vi "Test FPGA.vi"() -> ()   [LabVIEW 2014]
uses:
  <vilib>/FPGAPlugInAG/PXI-7842R/niLvFpga_Open_PXI-7842R.vi
  <vilib>/rvi/interface/common/dynamic/niFpgaDynamicAddResources.vi
  <vilib>/rvi/interface/common/niFpgaWaitOnOcc.vi
  <vilib>/Utility/error.llb/Error Cluster From Error Code.vi
  <vilib>/rvi/errors/niLvFpgaAdjustHostInterfaceError.vi
  <vilib>/RVI Host/nirviSupport.llb/nirviErrorClusterFromErrorCode.vi
  <vilib>/FPGAPlugInAG/Dynamic/niLvFpga_Close_Dynamic.vi
  <vilib>/rvi/interface/nirviOpenFPGA/nirviOpenFPGA.xnode
  FPGA Bitfiles/FPGA Server.lvbitx
  <vilib>/rvi/interface/nirviMethod/nirviMethod.xnode
  <vilib>/rvi/interface/nirviReadWriteControl/nirviReadWriteControl.xnode
  <vilib>/rvi/interface/nirviCloseFPGA/nirviCloseFPGA.xnode
  <vilib>/FPGAPlugInAG/Dynamic/niLvFpga_ConfigureFifo_Dynamic.vi
  <vilib>/rvi/errors/niLvFpgaMergeErrorWithErrorCode.vi
  NiFpgaLv.dll
  <vilib>/rvi/interface/Simulation/niFpgaSimulationCallBeginRW.vi
  <vilib>/FPGAPlugInAG/Dynamic/niLvFpga_StartFifo_Dynamic.vi
  <vilib>/FPGAPlugInAG/Dynamic/niLvFpga_WriteFifo_Dynamic.vi
  <vilib>/FPGAPlugInAG/Dynamic/niLvFpga_ReadFifo_Dynamic.vi
  <vilib>/rvi/interface/nirviMethod/StockFPGA_InlinedMethodWaitForSingleIRQ.vi
  <vilib>/FPGAPlugInAG/Dynamic/niLvFpga_WaitOnIrq_Dynamic.vi
  <vilib>/FPGAPlugInAG/Dynamic/niLvFpga_AcknowledgeIrq_Dynamic.vi
panel:
  in  "iSpk Enable":T1
  in  "LaserEn":T1
  out "Waveform Graph":i16[](graph)
  in  "Speaker":cluster{"Voltage":fxp<+,32,0>, "Offset":i16} {"Voltage" format="%.32g"}
  out "error out 2":errorcluster
  out "error out":errorcluster
  out "current time":timestamp
  out "Elements Remaining":u32
  in  "f0":i16=1350
  in  "Df":i16=200
  in  "Spk Enable":bool
  in  "Cell 5":T2 {"f0" format="%.32g"; "Scale" format="%.32g"}
  in  "Stop Button":bool
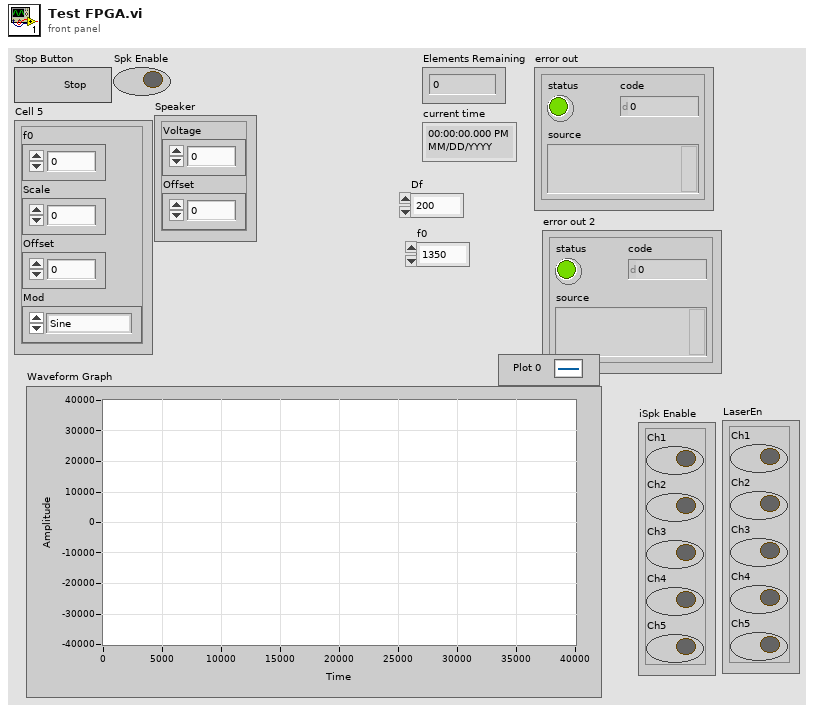
[diagram p1: front panel]
types:
  T1 = cluster{"Ch1":bool, "Ch2":bool, "Ch3":bool, "Ch4":bool, "Ch5":bool}
  T2 = cluster{"f0":fxp<+,32,0>, "Scale":fxp<+,32,0>, "Offset":i16, "Mod":enum8{"Sine", "Square"}}
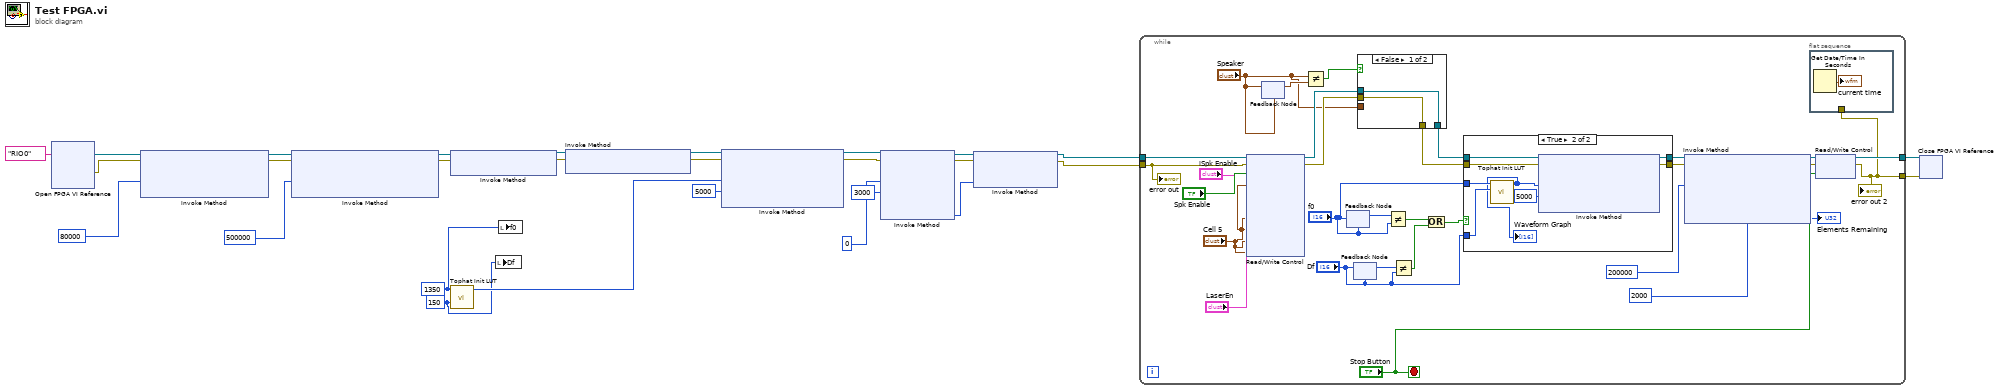
[diagram p0: block diagram]
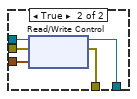
[diagram p2: hidden frame]
diagram:
  w13 = i16 150 ("Df")
  w14 = i16 1350 ("f0")
  n1 = xnode "Open FPGA VI Reference"("resource name"=tag "RIO0") -> ("FPGA VI Reference Out"=w27:refnum<k20>, "error out"=w23:errorcluster)  [unwired: 1 in]
  n2 = xnode "Invoke Method"("FPGA VI Reference In"=w27, "error in"=w23, "Requested Depth"=u32 80000) -> ("FPGA VI Reference Out"=w25:refnum<k20>, "error out"=w22:errorcluster)  [unwired: 1 out]
  n3 = xnode "Invoke Method"("FPGA VI Reference In"=w25, "error in"=w22, "Requested Depth"=u32 500000) -> ("FPGA VI Reference Out"=w21:refnum<k20>, "error out"=w20:errorcluster)  [unwired: 1 out]
  n4 = xnode "Invoke Method"("FPGA VI Reference In"=w21, "error in"=w20) -> ("FPGA VI Reference Out"=w19:refnum<k20>, "error out"=w18:errorcluster)
  n5 = call "Tophat Init LUT.vi"("Df"=w13, "f0"=w14) -> ("Init Data Out"=w15:i16[])  [unwired: 7 in]
  n6 = local write "Df"(w13) -> ()
  n7 = local write "f0"(w14) -> ()
  n8 = xnode "Invoke Method"("FPGA VI Reference In"=w19, "error in"=w18) -> ("FPGA VI Reference Out"=w17:refnum<k20>, "error out"=w16:errorcluster)
  n9 = xnode "Invoke Method"("FPGA VI Reference In"=w17, "error in"=w16, "Data"=w15, "Timeout (ms)"=5000) -> ("FPGA VI Reference Out"=w9:refnum<k20>, "error out"=w8:errorcluster)  [unwired: 1 out]
  n10 = xnode "Invoke Method"("FPGA VI Reference In"=w9, "error in"=w8, "IRQ Number(s)"=0, "Timeout (ms)"=3000) -> ("FPGA VI Reference Out"=w5:refnum<k20>, "error out"=w4:errorcluster, "IRQ(s) Asserted"=w3:i32)  [unwired: 1 out]
  n11 = xnode "Invoke Method"("FPGA VI Reference In"=w5, "error in"=w4, "IRQ Number(s)"=w3) -> ("FPGA VI Reference Out"=w2:refnum<k20>, "error out"=w1:errorcluster)
  n12 = while {
    tunnel: [w45] -> w11
    tunnel: [w41] -> w10
    tunnel: w2 -> [w40]
    tunnel: w1 -> [w39]
    stop <- "Stop Button" stop-if-true
    n13 = xnode "Read/Write Control"("FPGA VI Reference In"=w40, "error in"=w39, "Spk Enable"="Spk Enable", "Cell 5"="Cell 5", "iSpk Enable"="iSpk Enable", "LaserEn"="LaserEn", "Cell 4"="Cell 5", "Cell 3"="Cell 5", "Cell 2"="Cell 5", "Cell 1"="Cell 5") -> ("FPGA VI Reference Out"=w36:refnum<k20>, "error out"=w35:errorcluster)
    n14 = feedback-in #1("Speaker") -> ()
    n15 = feedback #1("Speaker") -> (w32:cluster{"Voltage":fxp<+,32,0>, "Offset":i16})
    n16 = Not Equal?(x="Speaker", y=w32) -> (x != y?=w31:bool)
    n17 = feedback-in #2("f0") -> ()
    n18 = feedback #2("f0") -> (w56:i16)
    n19 = feedback #3("Df") -> (w57:i16)
    n20 = feedback-in #3("Df") -> ()
    n21 = case shown="False" w31 {
      tunnel: w36 -> [w60 w65]
      tunnel: w35 -> [w59 w64]
      tunnel: [w60 w63] -> w34
      tunnel: [w59 w62] -> w33
      tunnel: "Speaker" -> [_ w61]
      frame False {
      }
      frame True {
        n22 = xnode "Read/Write Control"("FPGA VI Reference In"=w65, "error in"=w64, "Speaker"=w61) -> ("FPGA VI Reference Out"=w63:refnum<k20>, "error out"=w62:errorcluster)
      }
    }
    n23 = Not Equal?(x=w56, y="f0") -> (x != y?=w55:bool)
    n24 = Not Equal?(x=w57, y="Df") -> (x != y?=w54:bool)
    n25 = Or(x=w55, y=w54) -> (x .or. y?=w53:bool)
    n26 = case shown="True" w53 {
      tunnel: "f0" -> [_ w76]
      tunnel: "Df" -> [_ w75]
      tunnel: w34 -> [w68 w74]
      tunnel: w33 -> [w67 w73]
      tunnel: [w68 w72] -> w50
      tunnel: [w67 w71] -> w49
      frame False {
      }
      frame True {
        n27 = call "Tophat Init LUT.vi"("Df"=w75, "f0"=w76) -> ("Init Data Out"=w69:i16[])  [unwired: 7 in]
        "Waveform Graph" <- w69
        n28 = xnode "Invoke Method"("FPGA VI Reference In"=w74, "error in"=w73, "Data"=w69, "Timeout (ms)"=5000) -> ("FPGA VI Reference Out"=w72:refnum<k20>, "error out"=w71:errorcluster)  [unwired: 1 out]
      }
    }
    n29 = xnode "Invoke Method"("FPGA VI Reference In"=w50, "error in"=w49, "Number of Elements"=u32 200000, "Timeout (ms)"=2000) -> ("FPGA VI Reference Out"=w48:refnum<k20>, "error out"=w47:errorcluster, "Elements Remaining"=→"Elements Remaining":u32)  [unwired: 1 out]
    n30 = flat-sequence {
      tunnel: w41 -> [_]
      frame #0 {
        n31 = Get Date/Time In Seconds() -> (seconds since 1Jan1904=→"current time":timestamp)
      }
    }
    n32 = xnode "Read/Write Control"("FPGA VI Reference In"=w48, "error in"=w47, "stop"="Stop Button") -> ("FPGA VI Reference Out"=w45:refnum<k20>, "error out"=w41:errorcluster)
    "error out 2" <- w41
    "error out" <- w39
  }
  n33 = xnode "Close FPGA VI Reference"("FPGA VI Reference In"=w11, "error in"=w10) -> ()  [unwired: 1 out]
